vi "Set Action Current Arrays.vi"(6 "Direction":T1, 7 "Team Index":i32, 8 "Action":T2, 9 "Column":i32, 10 "Row":i32, 11 "MoveTrack":i32[][](array[numeric])) -> (3 "MoveTrack Out":i32[][](array[numeric]))   [LabVIEW 2016, in "AntFarm_MB.lvclass"]
uses:
  AntFarm_MB.lvclass
  Type Defs/Action Enum.ctl
  Type Defs/Direction Enum.ctl
  Type Defs/SB Type Defs.lvlib
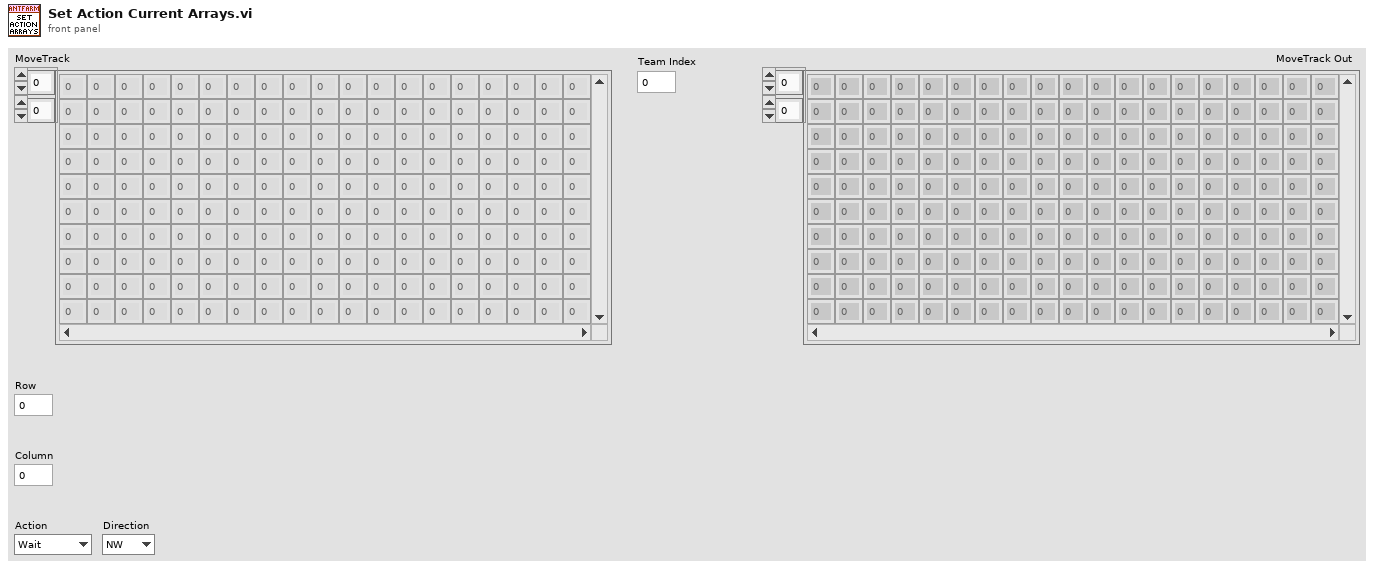
[diagram p1: front panel]
types:
  T1 = typedef "SB Type Defs.lvlib/Direction Enum.ctl" = enum16{"NW", "N", "NE", "E", "SE", "S", "SW", "W"}
  T2 = typedef "SB Type Defs.lvlib/Action Enum.ctl" = enum16{"Wait", "Move", "Attack", "Replicate"}
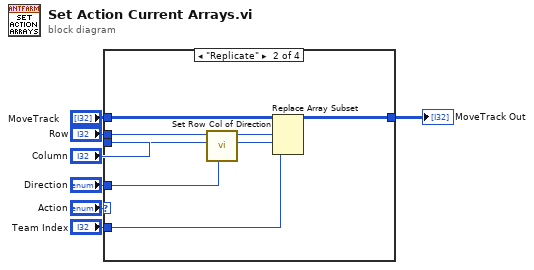
[diagram p0: block diagram]
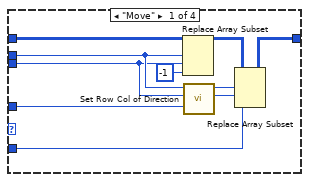
[diagram p2: hidden frame]
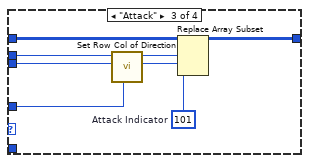
[diagram p3: hidden frame]
diagram:
  n1 = case shown="\"Replicate\"" "Action" {
    tunnel: "Direction" -> [w9 w19 w26 _]
    tunnel: "Column" -> [w10 w24 w32 _]
    tunnel: "Row" -> [w11 w23 w31 _]
    tunnel: "MoveTrack" -> [w17 w20 w27 w34]
    tunnel: [w15 w25 w33 w34] -> w3
    tunnel: "Team Index" -> [w8 w18 _ _]
    frame "Move" {
      n2 = Replace Array Subset(array=w17, new element=-1 ("new element/subarray"), index (row)=w11, index (col)=w10) -> (w16:i32[][])
      n3 = call "Set Row Col of Direction.vi"("Direction"=w9, "Column"=w10, "Row"=w11) -> ("Col Direction"=w13:i32, "Row Direction"=w14:i32)  [unwired: 7 in]
      n4 = Replace Array Subset(array=w16, new element=w8, index (row)=w14, index (col)=w13) -> (w15:i32[][])
    }
    frame "Replicate" {
      n5 = call "Set Row Col of Direction.vi"("Direction"=w19, "Column"=w24, "Row"=w23) -> ("Col Direction"=w21:i32, "Row Direction"=w22:i32)  [unwired: 7 in]
      n6 = Replace Array Subset(array=w20, new element=w18, index (row)=w22, index (col)=w21) -> (w25:i32[][])
    }
    frame "Attack" {
      w28 = 101  # Attack Indicator
      n7 = call "Set Row Col of Direction.vi"("Direction"=w26, "Column"=w32, "Row"=w31) -> ("Col Direction"=w29:i32, "Row Direction"=w30:i32)  [unwired: 7 in]
      n8 = Replace Array Subset(array=w27, new element=w28, index (row)=w30, index (col)=w29) -> (w33:i32[][])
    }
    frame "Wait" {
    }
  }
  "MoveTrack Out" <- w3
